vi "Replace Missing Items in Hierarchy Test.vi"() -> (2 "Result":bool)   [LabVIEW 2014, in "SystemConfigReop Tests.lvlib"]
uses:
  SystemConfigReop Tests.lvlib
  <vilib>/NI/Configuration Framework/class discovery singleton/class discovery singleton methods.ctl
  <vilib>/NI/Configuration Framework/tree serializer/flat hierarchy.ctl
  <vilib>/NI/Configuration Framework/tree serializer/full hierarchy.ctl
  <vilib>/NI/Configuration Framework/tree serializer/hierarchy element.ctl
  <vilib>/NI/Configuration Framework/tree serializer/instance data.ctl
  Configuration Editor/Classes/SystemConfigRepo/SystemConfigRepo.lvclass
  <vilib>/NI/Configuration Framework/tree serializer/NISE_CEF_TreeSerializer.lvlib
  <vilib>/NI/Configuration Framework/class discovery singleton/class discovery singleton.lvlib
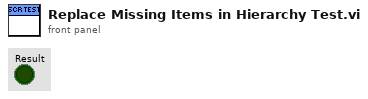
[diagram p1: front panel]
types:
  T1 = typedef "class discovery singleton.lvlib/class discovery singleton methods.ctl" = enum16{"add search paths", "load class by name", "list available classes", "get class path", "delete cache"}
  T2 = typedef "NISE_CEF_TreeSerializer.lvlib/flat hierarchy.ctl" = cluster{"hierarchy structure":T3, "instance data":T5[]}
  T3 = typedef "NISE_CEF_TreeSerializer.lvlib/full hierarchy.ctl" = cluster{"root":string, "hierarchy":T4[]}
  T4 = typedef "NISE_CEF_TreeSerializer.lvlib/hierarchy element.ctl" = cluster{"current node":string, "children":string[]}
  T5 = typedef "NISE_CEF_TreeSerializer.lvlib/instance data.ctl" = cluster{"ID":string, "Alias":string, "class":string, "version":string, "data":string}
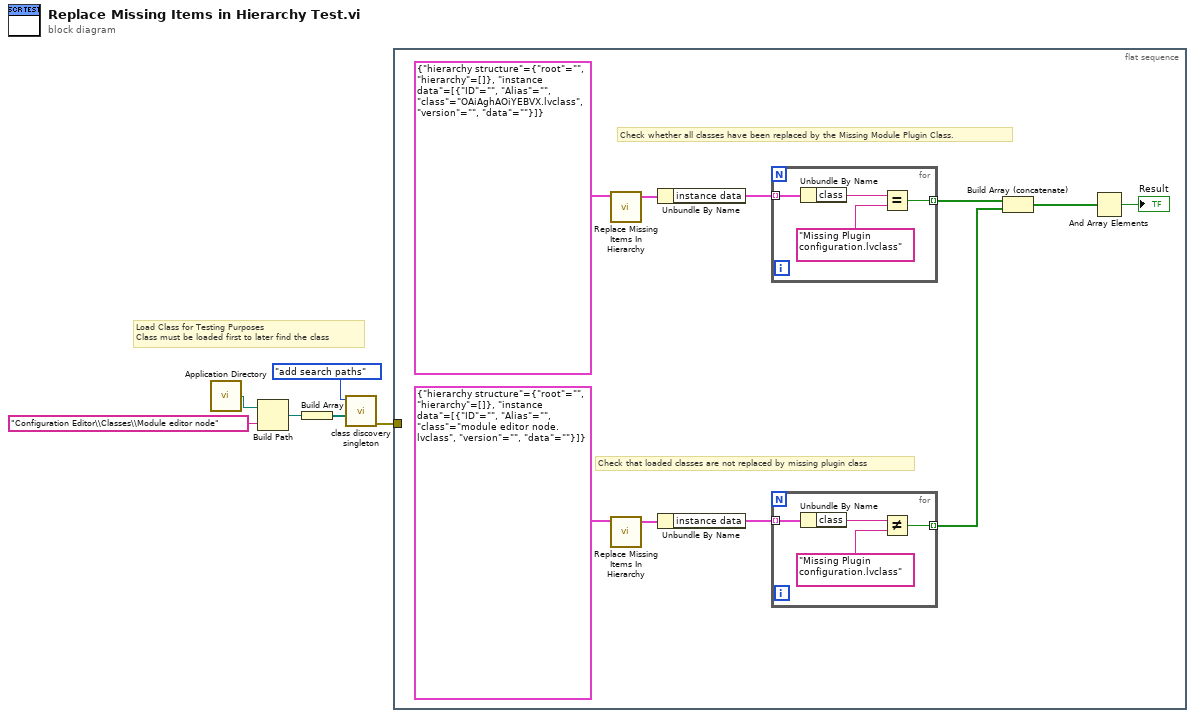
[diagram p0: block diagram]
diagram:
  # "Load Class for Testing Purposes\nClass must be loaded first to later find the class"
  n1 = call <vilib>:"Application Directory.vi"() -> ("Application Directory"=w5:path)
  n2 = Build Path(base path=w5, name or relative path="Configuration Editor\\Classes\\Module editor node") -> (appended path=w3:path)
  n3 = Build Array(w3) -> (w2:path[])
  n4 = call <vilib>:"class discovery singleton.vi"("Plugin Search Paths"=w2, "method"=class_discovery_singleton_methods."add search paths") -> ("error out"=w1:errorcluster)  [unwired: 6 in, 3 out]
  n5 = flat-sequence {
    tunnel: w1 -> [_]
    frame #0 {
      # "Check that loaded classes are not replaced by missing plugin class"
      # "Check whether all classes have been replaced by the Missing Module Plugin Class."
      n6 = call "Replace Missing Items In Hierarchy.vi"("Flat Hierarchy"=T2 {"hierarchy structure"={"root"="", "hierarchy"=[]}, "instance data"=[{"ID"="", "Alias"="", "class"="OAiAghAOiYEBVX.lvclass", "version"="", "data"=""}]}) -> ("Flat Hierarchy"=w15:T2)  [unwired: 10 in]
      n7 = call "Replace Missing Items In Hierarchy.vi"("Flat Hierarchy"=T2 {"hierarchy structure"={"root"="", "hierarchy"=[]}, "instance data"=[{"ID"="", "Alias"="", "class"="module editor node.lvclass", "version"="", "data"=""}]}) -> ("Flat Hierarchy"=w10:T2)  [unwired: 10 in]
      n8 = Unbundle By Name(w15) -> ("instance data"=w14:T5[])
      n9 = Unbundle By Name(w10) -> ("instance data"=w11:T5[])
      n10 = for {
        tunnel: w14 -> [w24] mode=indexing
        tunnel: [w21] -> w13 mode=indexing
        n11 = Unbundle By Name(w24) -> ("class"=w23:string)
        n12 = Equal?(x=w23, y="Missing Plugin configuration.lvclass") -> (x = y?=w21:bool)
      }
      n13 = for {
        tunnel: w11 -> [w20] mode=indexing
        tunnel: [w17] -> w7 mode=indexing
        n14 = Unbundle By Name(w20) -> ("class"=w19:string)
        n15 = Not Equal?(x=w19, y="Missing Plugin configuration.lvclass") -> (x != y?=w17:bool)
      }
      n16 = Build Array (concatenate)(w13, w7) -> (w8:bool[])
      n17 = And Array Elements(Boolean array=w8) -> (logical AND=→"Result":bool)
    }
  }
